vi "startEncoder.vi"(1 "MXP Port":enum16{"A", "B"}(ring)) -> (0 "SPI Config Out":T1)   [LabVIEW 2019]
uses:
  SPI/SPI Config.ctl
panel:
  in  "SPI Config":T1
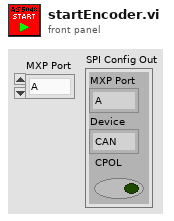
[diagram p1: front panel]
types:
  T1 = typedef "SPI Config.ctl" = cluster{"MXP Port":enum16{"A", "B"}, "Device":enum16{"CAN", "ENC", "IMU1", "IMU2"}, "CPOL":bool}
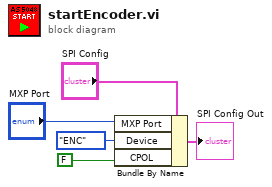
[diagram p0: block diagram]
diagram:
  n1 = Bundle By Name(cluster="SPI Config", "MXP Port"="MXP Port", "Device"=enum16{"CAN", "ENC", "IMU1", "IMU2"}."ENC", "CPOL"=FALSE) -> (→"SPI Config Out":T1)
